vi "Rinocloud_navigation_panel.vi"(7 "metadata":T1 {"custom metadata array"."Data type" items=["Numeric", "String", "1D array of strings", "1D array of doubles", "Data JSON string", "<null>"]}, 8 "active directory ID":string, 9 "new folder ref":refnum<vi>, 10 "ancestor tree ref":refnum<vi>, 11 "children tree ref":refnum<vi>) -> (3 "active items":T2)   [LabVIEW 2013]
uses:
  Rinocloud Library.lvlib
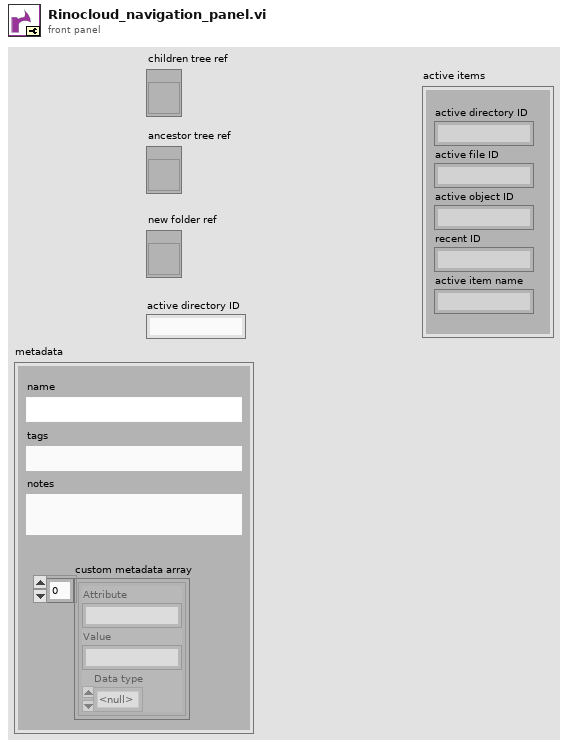
[diagram p1: front panel]
types:
  T1 = cluster{"name":string, "tags":string, "notes":string, "custom metadata array":cluster{"Attribute":string, "Value":string, "Data type":u16}[]}
  T2 = cluster{"active directory ID":string, "active file ID":string, "active object ID":string, "recent ID":string, "active item name":string}
  T3 = cluster{"Attribute":string, "Value":string, "Data type":u16}[]
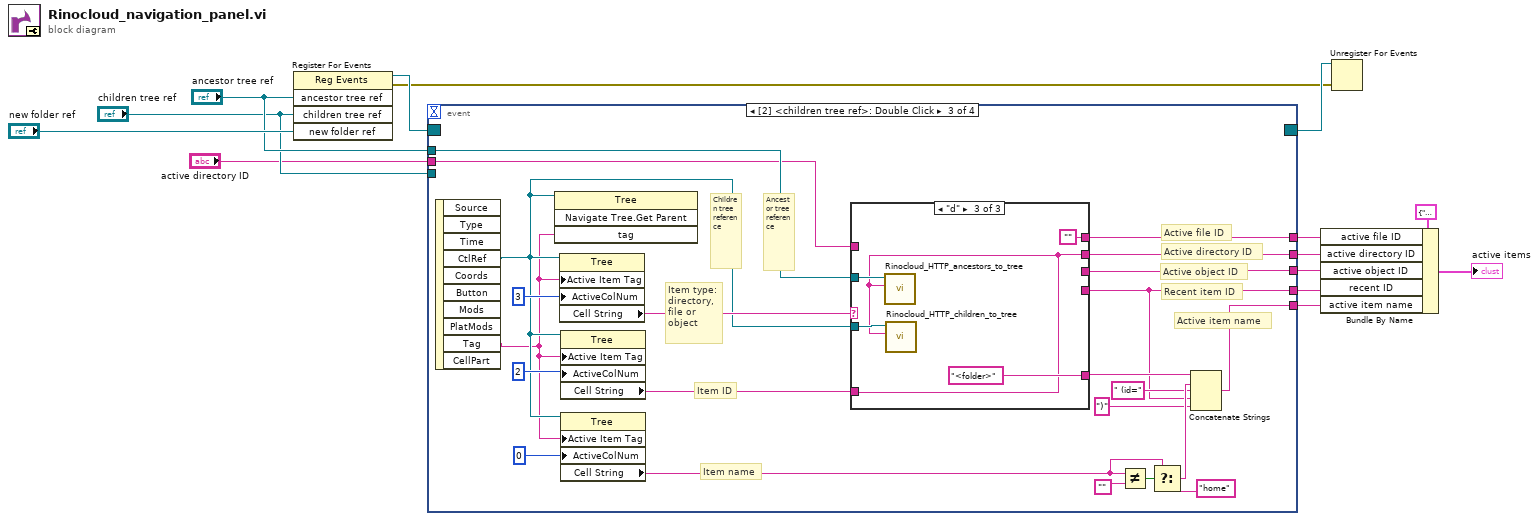
[diagram p0: block diagram]
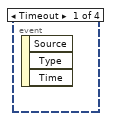
[diagram p2: hidden frame]
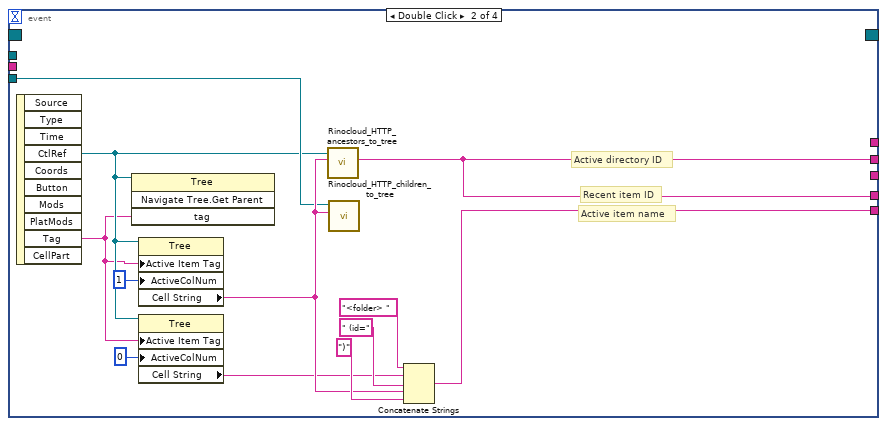
[diagram p3: hidden frame]
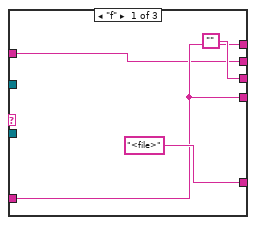
[diagram p4: hidden frame]
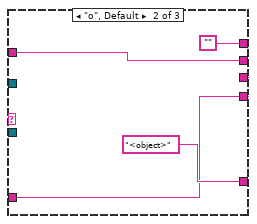
[diagram p5: hidden frame]
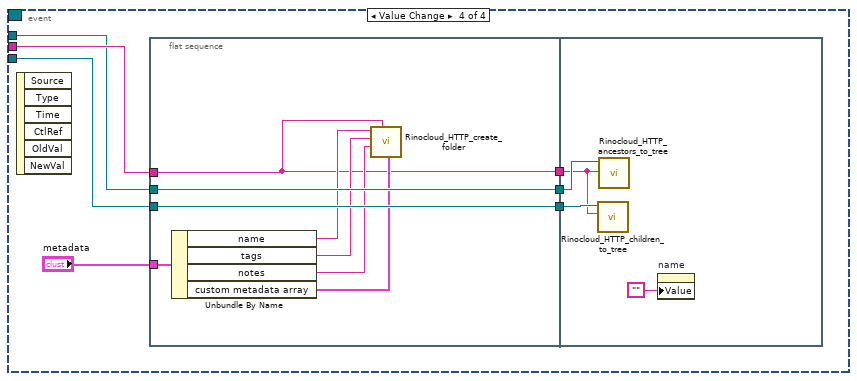
[diagram p6: hidden frame]
diagram:
  n1 = register-events("ancestor tree ref", "children tree ref", "new folder ref") -> (reference out=w14:refnum<event-registration>, error out=w12:errorcluster)  [unwired: 2 in]
  n2 = event shown="[2] <children tree ref>: Double Click" {
    selector: w14 -> [_ _ _ _]
    dyn-events: [_ _ _ _] -> w13
    timeout: _ -> [_ _ _ _]
    tunnel: "ancestor tree ref" -> [_ _ w33 w64]
    tunnel: [_ _ w32 _] -> w8
    tunnel: [_ w15 w31 _] -> w7
    tunnel: [_ _ w30 _] -> w6
    tunnel: [_ w15 w29 _] -> w5
    tunnel: [_ w16 w28 _] -> w4
    tunnel: "children tree ref" -> [_ w19 _ w63]
    tunnel: "active directory ID" -> [_ _ w27 w65]
    event Timeout {
      n3 = event-data() -> ()  [unwired: 1 in, 3 out]
    }
    event Double Click {
      # "Active item name"
      # "Recent item ID"
      # "Active directory ID"
      n4 = event-data() -> ("CtlRef"=w18:refnum<vi>, "Tag"=w17:string)  [unwired: 1 in, 8 out]
      n5 = invoke on="Invoke Node" class="Tree" method="Navigate Tree.Get Parent"(reference=w18, "tag"=w17) -> ()  [unwired: 2 in, 4 out]
      n6 = property on="Property Node" class="Tree"(reference=w18, "Active Item Tag"=w17, "ActiveColNum"=1 ("Active Cell:Active Column Number")) -> ("Cell String"=w21:string)  [unwired: 1 in, 2 out]
      n7 = property on="Property Node" class="Tree"(reference=w18, "Active Item Tag"=w17, "ActiveColNum"=0 ("Active Cell:Active Column Number")) -> ("Cell String"=w20:string)  [unwired: 1 in, 2 out]
      n8 = call "Rinocloud_HTTP_ancestors_to_tree.vi"("id"=w21, "Tree Ref in"=w18) -> ("last ID"=w15:string)  [unwired: 2 in, 3 out]
      n9 = call "Rinocloud_HTTP_children_to_tree.vi"("id"=w21, "Tree Ref in"=w19) -> ()  [unwired: 7 in, 3 out]
      n10 = Concatenate Strings("<folder> " ("string"), w20, " (id=" ("string"), w21, ")" ("string")) -> (w16:string)
    }
    event Double Click {
      # "Ancestor tree \nreference"
      # "Children tree \nreference"
      # "Item name"
      # "Item type:\ndirectory,\nfile or\nobject"
      # "Item ID"
      # "Active item name"
      # "Recent item ID"
      # "Active object ID"
      # "Active directory ID"
      # "Active file ID"
      n11 = event-data() -> ("CtlRef"=w35:refnum<vi>, "Tag"=w34:string)  [unwired: 1 in, 8 out]
      n12 = invoke on="Invoke Node" class="Tree" method="Navigate Tree.Get Parent"(reference=w35, "tag"=w34) -> ()  [unwired: 2 in, 4 out]
      n13 = property on="Property Node" class="Tree"(reference=w35, "Active Item Tag"=w34, "ActiveColNum"=3 ("Active Cell:Active Column Number")) -> ("Cell String"=w38:string)  [unwired: 1 in, 2 out]
      n14 = property on="Property Node" class="Tree"(reference=w35, "Active Item Tag"=w34, "ActiveColNum"=2 ("Active Cell:Active Column Number")) -> ("Cell String"=w37:string)  [unwired: 1 in, 2 out]
      n15 = property on="Property Node" class="Tree"(reference=w35, "Active Item Tag"=w34, "ActiveColNum"=0 ("Active Cell:Active Column Number")) -> ("Cell String"=w36:string)  [unwired: 1 in, 2 out]
      n16 = case shown="\"d\"" w38 {
        tunnel: w37 -> [w50 w55 w57]
        tunnel: ["<file>" ("f") "<object>" ("f") "<folder>" ("f")] -> w45
        tunnel: [w50 w55 w57] -> w29
        tunnel: ["" w55 w60] -> w30
        tunnel: [w50 "" w60] -> w32
        tunnel: [w49 w53 w57] -> w31
        tunnel: w33 -> [_ _ w59]
        tunnel: w35 -> [_ _ w58]
        tunnel: w27 -> [w49 w53 _]
        frame "f" {
        }
        frame "o", Default {
        }
        frame "d" {
          w60 = ""
          n17 = call "Rinocloud_HTTP_ancestors_to_tree.vi"("id"=w57, "Tree Ref in"=w59) -> ()  [unwired: 2 in, 4 out]
          n18 = call "Rinocloud_HTTP_children_to_tree.vi"("id"=w57, "Tree Ref in"=w58) -> ()  [unwired: 7 in, 3 out]
        }
      }
      n19 = Not Equal?(x=w36, y="") -> (x != y?=w47:bool)
      n20 = Select(t=w36, s=w47, f="home") -> (s? t:f=w44:string)
      n21 = Concatenate Strings(w45, w44, " (id=" ("string"), w29, ")" ("string")) -> (w28:string)
    }
    event Value Change {
      n22 = event-data() -> ()  [unwired: 1 in, 6 out]
      n23 = flat-sequence {
        tunnel: w65 -> [w69]
        tunnel: w64 -> [w76]
        tunnel: w63 -> [w75]
        tunnel: [w69] -> w68
        tunnel: [w76] -> w67
        tunnel: [w75] -> w66
        tunnel: "metadata" -> [w74]
        tunnel: w68 -> [w77]
        tunnel: w67 -> [w79]
        tunnel: w66 -> [w78]
        frame #0 {
          n24 = Unbundle By Name(w74) -> ("name"=w70:string, "tags"=w71:string, "notes"=w72:string, "custom metadata array"=w73:T3)
          n25 = call "Rinocloud_HTTP_create_folder.vi"("Extra metadata array"=w73, "Parent ID"=w69, "Notes"=w72, "Tags"=w71, "Name"=w70) -> ()  [unwired: 3 in, 2 out]
        }
        frame #1 {
          n26 = call "Rinocloud_HTTP_children_to_tree.vi"("id"=w77, "Tree Ref in"=w78) -> ()  [unwired: 7 in, 3 out]
          n27 = call "Rinocloud_HTTP_ancestors_to_tree.vi"("id"=w77, "Tree Ref in"=w79) -> ()  [unwired: 2 in, 4 out]
          n28 = property on="name" class="Str"("Value"="") -> ()  [unwired: 2 in, 2 out]
        }
      }
    }
  }
  n29 = Bundle By Name(cluster=T2 {"active directory ID"="", "active file ID"="", "active object ID"="", "recent ID"="", "active item name"=""} ("active items 2"), "active file ID"=w8, "active directory ID"=w7, "active object ID"=w6, "recent ID"=w5, "active item name"=w4) -> (→"active items":T2)
  n30 = Unregister For Events(event registration refnum=w13, error in=w12) -> ()  [unwired: 1 out]
